vi "Create AIs RT FIFO.vi"(8 "error in":errorcluster) -> (0 "error out":errorcluster, 3 "AIs RT FIFO out":refnum<k33>)   [LabVIEW 2021, in "RT Main.lvlib"]
uses:
  RT Main.lvlib
  Libraries/Common Files/Common Files.lvlib
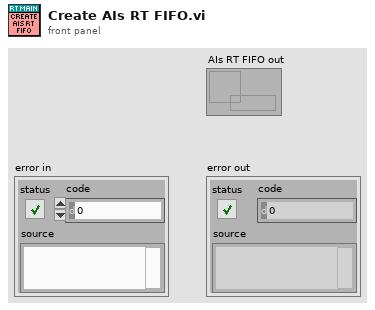
[diagram p1: front panel]
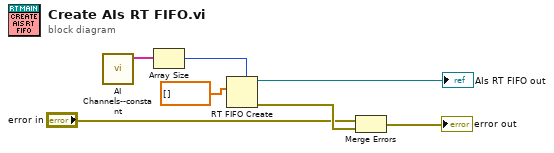
[diagram p0: block diagram]
diagram:
  n1 = call "AI Channels--constant.vi"() -> ("AI Channels"=w7:tag[])  [unwired: 11 in]
  n2 = Array Size(array=w7) -> (size(s)=w1:i32)
  n3 = RT FIFO Create(1:sgl[] [], 6:w1) -> (8:→"AIs RT FIFO out":refnum<k33>, 11:w6:errorcluster)  [unwired: 6 in, 1 out]
  n4 = Merge Errors("error in", w6) -> (→"error out":errorcluster)
